vi "Module - RH_MALING.vi"() -> ()   [LabVIEW 2019]
uses:
  Control/State - eFGV.ctl
panel:
  out "Site Name":string="RH MALING (7.28 kWp)"
  out "BANK-02-TEMP":dbl caption="T_bat" format="%#_g C"
  out "BANK-02-IDC":dbl caption="I_bat" format="%.2f A"
  out "BANK-02-VDC":dbl caption="V_bat" format="%.1f V"
  out "BANK-02-SOC":dbl caption="SOC" format="%#_g %"
  out "PM-01-STATUS":bool
  out "PM-01-FREQ":dbl caption="Freq" format="%.0f Hz"
  out "PM-01-IAC":dbl caption="Iac" format="%.0f A"
  out "PM-01-VAC":dbl caption="Vac" format="%.0f V"
  out "PM-01-PAC":dbl caption="Pac" format="%.0f W"
  out "SI-M-01-STATUS":bool
  out "SI-M-01-FREQ":dbl caption="FREQ" format="%.0f Hz"
  out "SI-M-01-L3":dbl caption="L3" format="%.0f V"
  out "SI-M-01-L2":dbl caption="L2" format="%.0f V"
  out "SI-M-01-L1":dbl caption="L1" format="%.0f V"
  out "SI-M-01-PAC":dbl caption="Pac" format="%.0f W"
  out "BANK-01-TEMP":dbl caption="T_bat" format="%#_g C"
  out "BANK-01-IDC":dbl caption="I_bat" format="%.2f A"
  out "BANK-01-VDC":dbl caption="V_bat" format="%.1f V"
  out "BANK-01-SOC":dbl caption="SOC" format="%#_g %"
  out "SB-02-STATUS":bool
  out "SB-02-A-IDC":dbl caption="A.Idc" format="%.1f A"
  out "SB-02-A-VDC":dbl caption="A.Vdc" format="%.0f V"
  out "SB-02-PAC":dbl caption="Pac" format="%#_g W"
  out "SB-01-STATUS":bool
  out "SB-01-A-IDC":dbl caption="A.Idc" format="%.1f A"
  out "SB-01-A-VDC":dbl caption="A.Vdc" format="%.0f V"
  out "SB-01-PAC":dbl caption="Pac" format="%.0f W"
  # "RH MALING (7.28 kWp)"
  # "SB-01"
  # "SB-02"
  # "BANK-2"
  # "PM-01"
  # "SI"
  # "BANK-1"
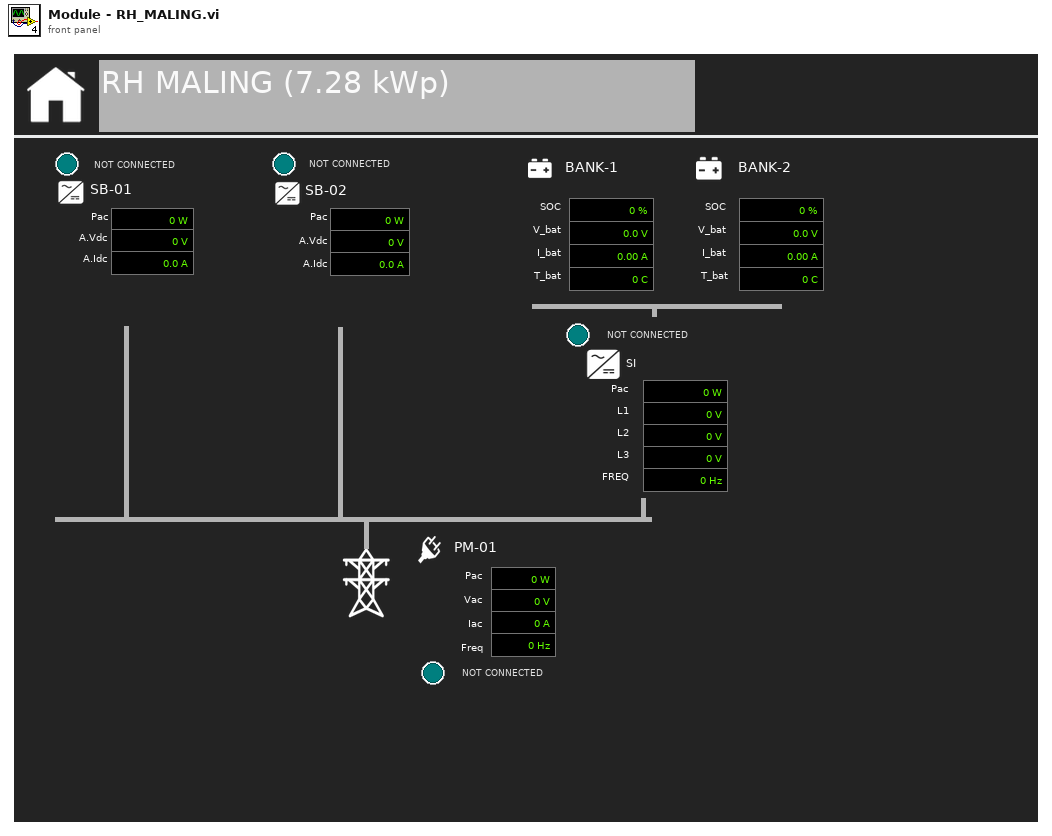
[diagram p1: front panel]
types:
  T1 = typedef "State - eFGV.ctl" = enum16{"Init", "Read", "Write", "Close"}
  T2 = typedef "Device Name.ctl" = enum16{"SB-01", "SB-02", "SB-03", "SB-04", "STP-01", "STP-02", "STP-03", "STP-04", "BANK-01", "BANK-02", "BANK-03", "BANK-04", "SI-M-01", "SI-M-02", "SI-M-03", "SI-M-04", "PM-01", "PM-02", "PM-03", "PM-04"}
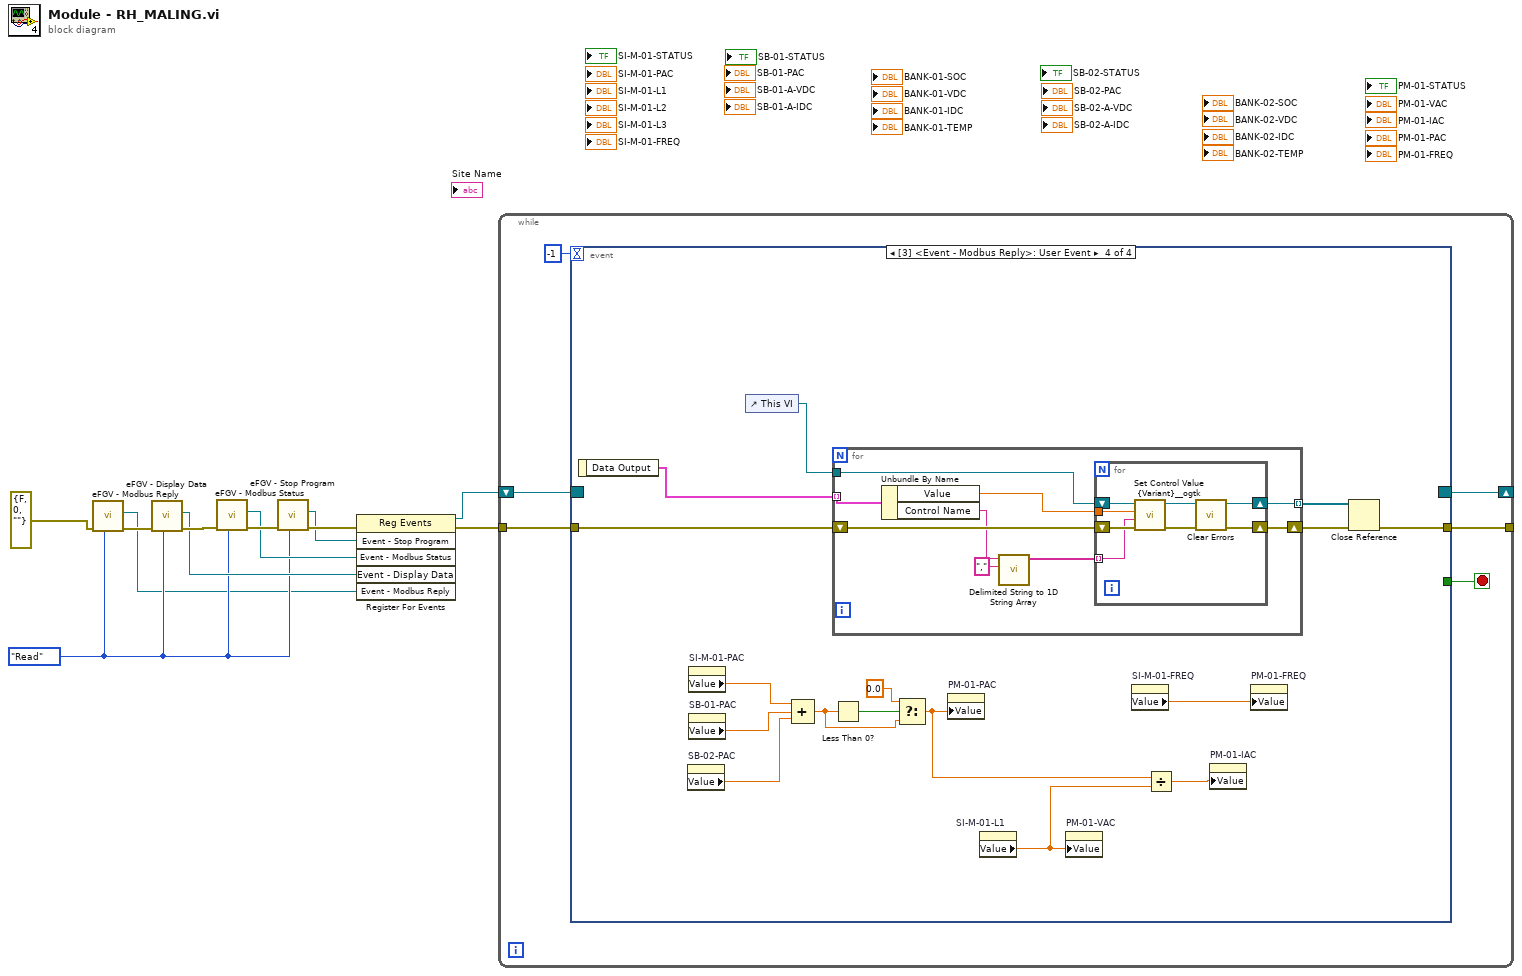
[diagram p0: block diagram]
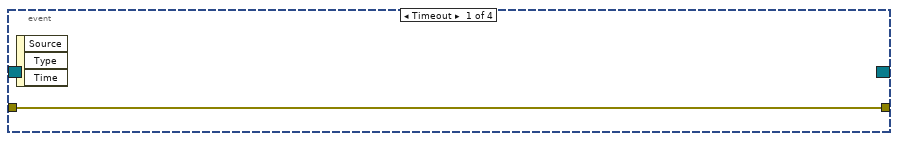
[diagram p2: hidden frame]
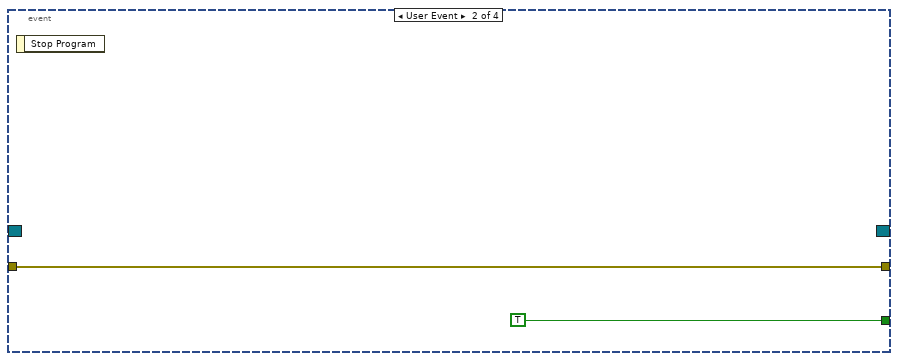
[diagram p3: hidden frame]
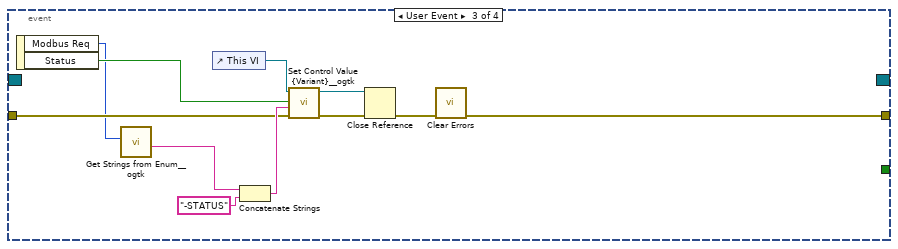
[diagram p4: hidden frame]
diagram:
  w2 = State_-_eFGV."Read" ("State - eFGV")
  n1 = call "eFGV - Modbus Reply.vi"("State - eFGV"=w2, "error in (no error)"=errorcluster {"status"=FALSE, "code"=0, "source"=""}) -> ("error out"=w4:errorcluster, "Event - Modbus Reply"=w1:refnum<user-event>)  [unwired: 8 in]
  n2 = call "eFGV - Display Data.vi"("State - eFGV"=w2, "error in (no error)"=w4) -> ("error out"=w6:errorcluster, "Event - Display Data"=w5:refnum<user-event>)  [unwired: 8 in]
  n3 = call "eFGV - Modbus Status.vi"("State - eFGV"=w2, "error in (no error)"=w6) -> ("error out"=w8:errorcluster, "Event - Modbus Status"=w7:refnum<user-event>)  [unwired: 8 in]
  n4 = call "eFGV - Stop Program.vi"("State - eFGV"=w2, "error in (no error)"=w8) -> ("error out"=w11:errorcluster, "Event - Stop Program"=w10:refnum<user-event>)  [unwired: 8 in]
  n5 = register-events(error in=w11, w10, w7, w5, w1) -> (reference out=w9:refnum<event-registration>, error out=w12:errorcluster)  [unwired: 1 in]
  n6 = while {
    tunnel: w12 -> [w17]
    shift-right: [w16] -> _
    shift-left: w9 -> [w18]
    tunnel: [w13] -> _
    stop <- w15 stop-if-true
    n7 = event shown="[3] <Event - Modbus Reply>: User Event" {
      selector: w18 -> [_ _ _ _]
      dyn-events: [_ _ _ _] -> w16
      timeout: -1 -> [_ _ _ _]
      tunnel: w17 -> [w19 w20 w30 w47]
      tunnel: [_ TRUE _ _] -> w15
      tunnel: [w19 w20 w22 w43] -> w13
      event Timeout {
        n8 = event-data() -> ()  [unwired: 1 in, 3 out]
      }
      event User Event {
        n9 = event-data() -> ()  [unwired: 1 in, 1 out]
      }
      event User Event {
        n10 = event-data() -> ("Modbus Req"=w25:T2, "Status"=w29:bool)  [unwired: 1 in]
        n11 = call "Get Strings from Enum__ogtk.vi"("Enum"=w25) -> ("String Value"=w24:string)  [unwired: 7 in, 3 out]
        n12 = control-ref of="This VI"() -> (w32:refnum<vi>)
        n13 = Concatenate Strings(w24, "-STATUS" ("string")) -> (w31:string)
        n14 = call "Set Control Value {Variant}__ogtk.vi"("error in (no error)"=w30, "Control Name (\"\": use variant name)"=w31, "Value"=w29, "VI Refnum"=w32) -> ("error out"=w28:errorcluster, "VI Refnum dup"=w26:refnum<vi>)  [unwired: 6 in]
        n15 = Close Reference(reference=w26, error in (no error)=w28) -> (error out=w27:errorcluster)
        n16 = call <vilib>:"Clear Errors.vi"("error in (no error)"=w27) -> ("error out"=w22:errorcluster)  [unwired: 5 in, 1 out]
      }
      event User Event {
        n17 = event-data() -> ("Data Output"=w44:cluster{"Control Name":string, "Value":dbl}[])  [unwired: 1 in]
        n18 = property on="SB-02-PAC" class="DigNum (strict)"() -> ("Value"=w39:dbl)  [unwired: 2 in, 2 out]
        n19 = property on="SI-M-01-PAC" class="DigNum (strict)"() -> ("Value"=w41:dbl)  [unwired: 2 in, 2 out]
        n20 = property on="SB-01-PAC" class="DigNum (strict)"() -> ("Value"=w40:dbl)  [unwired: 2 in, 2 out]
        n21 = control-ref of="This VI"() -> (w48:refnum<vi>)
        n22 = Compound Arithmetic op=ADD(w41, w40, w39) -> (w37:dbl)
        n23 = for {
          tunnel: w48 -> [w57]
          tunnel: [w54] -> w45 mode=indexing
          tunnel: w44 -> [w53] mode=indexing
          shift-right: [w55] -> w46
          shift-left: w47 -> [w56]
          n24 = Unbundle By Name(w53) -> ("Value"=w52:dbl, "Control Name"=w51:string)
          n25 = call <vilib>:"Delimited String to 1D String Array.vi"("delimiter"=",", "delimited string"=w51) -> ("string array"=w49:string[])  [unwired: 9 in]
          n26 = for {
            tunnel: w52 -> [w60]
            shift-right: [w61] -> w54
            shift-left: w57 -> [w64]
            shift-right: [w58] -> w55
            shift-left: w56 -> [w63]
            tunnel: w49 -> [w59] mode=indexing
            n27 = call "Set Control Value {Variant}__ogtk.vi"("error in (no error)"=w63, "Control Name (\"\": use variant name)"=w59, "Value"=w60, "VI Refnum"=w64) -> ("error out"=w62:errorcluster, "VI Refnum dup"=w61:refnum<vi>)  [unwired: 6 in]
            n28 = call <vilib>:"Clear Errors.vi"("error in (no error)"=w62) -> ("error out"=w58:errorcluster)  [unwired: 5 in, 1 out]
          }
        }
        n29 = Less Than 0?(x=w37) -> (x < 0?=w38:bool)
        n30 = Select(t=0.0, s=w38, f=w37) -> (s? t:f=w34:dbl)
        n31 = property on="PM-01-PAC" class="DigNum (strict)"("Value"=w34) -> ()  [unwired: 2 in, 2 out]
        n32 = property on="SI-M-01-L1" class="DigNum (strict)"() -> ("Value"=w33:dbl)  [unwired: 2 in, 2 out]
        n33 = property on="PM-01-VAC" class="DigNum (strict)"("Value"=w33) -> ()  [unwired: 2 in, 2 out]
        n34 = property on="SI-M-01-FREQ" class="DigNum (strict)"() -> ("Value"=w42:dbl)  [unwired: 2 in, 2 out]
        n35 = Divide(x=w34, y=w33) -> (x/y=w35:dbl)
        n36 = property on="PM-01-IAC" class="DigNum (strict)"("Value"=w35) -> ()  [unwired: 2 in, 2 out]
        n37 = property on="PM-01-FREQ" class="DigNum (strict)"("Value"=w42) -> ()  [unwired: 2 in, 2 out]
        n38 = Close Reference(reference=w45, error in (no error)=w46) -> (error out=w43:errorcluster)
      }
    }
  }
